vi "Untitled 2.vi"() -> ()   [LabVIEW 2020]
uses:
  <vilib>/Instr/_visa.llb/VISA Configure Serial Port (Instr).vi
panel:
  in  "OK Button 2":bool
  in  "OK Button":bool
  in  "VISA resource name":refnum<visa-resource-name>
  in  "Boolean":bool
  in  "String 2":string
  out "String":string
  in  "Numeric":dbl
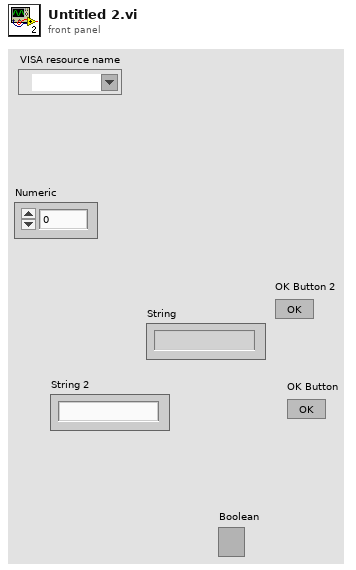
[diagram p1: front panel]
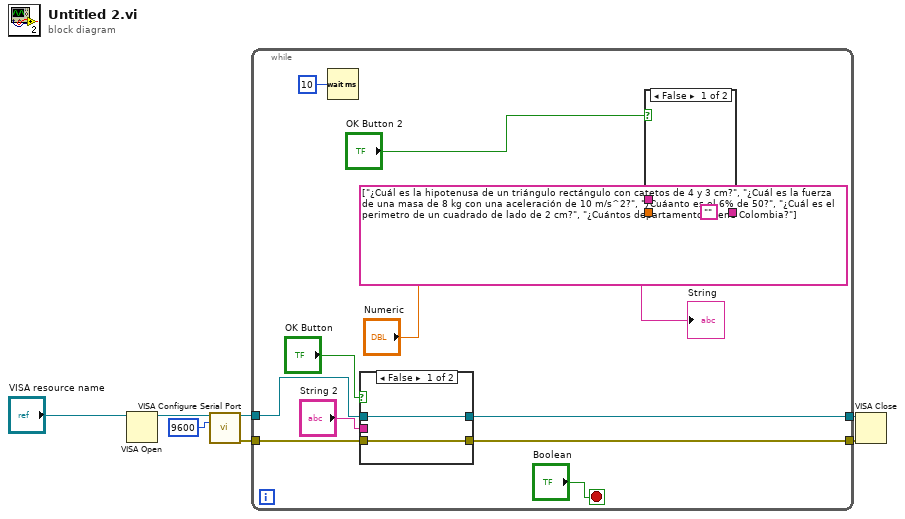
[diagram p0: block diagram]
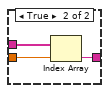
[diagram p2: hidden frame]
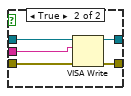
[diagram p3: hidden frame]
diagram:
  n1 = VISA Open(VISA resource name="VISA resource name") -> (VISA resource name=w7:refnum<visa-resource-name>)  [unwired: 4 in, 1 out]
  n2 = call-poly "VISA Configure Serial Port"("VISA resource name"=w7, "baud rate (9600)"=u32 9600) -> ("VISA resource name out"=w5:refnum<visa-resource-name>, "error out"=w4:errorcluster)  [unwired: 12 in]
  n3 = while {
    tunnel: w5 -> [w16]
    tunnel: w4 -> [w15]
    tunnel: [w14] -> w3
    tunnel: [w13] -> w2
    stop <- "Boolean" stop-if-true
    n4 = Wait (ms)(milliseconds to wait=u32 10) -> ()  [unwired: 1 out]
    n5 = case shown="False" "OK Button" {
      tunnel: w16 -> [w25 w30]
      tunnel: w15 -> [w24 w29]
      tunnel: [w25 w28] -> w14
      tunnel: [w24 w27] -> w13
      tunnel: "String 2" -> [_ w26]
      frame False {
      }
      frame True {
        n6 = VISA Write(VISA resource name=w30, write buffer=w26, error in (no error)=w29) -> (VISA resource name out=w28:refnum<visa-resource-name>, error out=w27:errorcluster)  [unwired: 1 out]
      }
    }
    n7 = case shown="False" "OK Button 2" {
      tunnel: string[] ["¿Cuál es la hipotenusa de un triángulo rectángulo con catetos de 4 y 3 cm?", "¿Cuál es la fuerza de una masa de 8 kg con una aceleración de 10 m/s^2?", "¿Cuáanto es el 6% de 50?", "¿Cuál es el perimetro de un cuadrado de lado de 2 cm?", "¿Cuántos departamentos tiene Colombia?"] ("Array") -> [_ w23]
      tunnel: "Numeric" -> [_ w22]
      tunnel: ["" w21] -> w17
      frame False {
      }
      frame True {
        n8 = Index Array(array=w23, index=w22) -> (element=w21:string)
      }
    }
    "String" <- w17
  }
  n9 = VISA Close(VISA resource name=w3, error in (no error)=w2) -> ()  [unwired: 1 out]
